vi "Anytime D Star Plan.vi"(6 "epsilon":dbl=1.0, 7 "overhaul (F)":bool, 8 "error in (no error)":errorcluster, 9 "new goal reference":refnum<data-value>, 10 "current reference":refnum<data-value>, 11 "Anytime D* in":refnum<class "NI_Robotics_AnytimeDStar.lvclass">) -> (0 "error out":errorcluster, 1 "no valid path exists":bool, 2 "path references":refnum<data-value>[](array[refnum]), 3 "Anytime D* out":refnum<class "NI_Robotics_AnytimeDStar.lvclass">, 4 "path cost":dbl)   [LabVIEW 2017, in "NI_Robotics_AnytimeDStar.lvclass"]
doc: "Plans a dynamic path through a map to the goal you specify. The first time this VI runs, the VI returns an initial path to a goal node within the map you specify in the Initialize AD* VI."
uses:
  <vilib>/robotics/Navigation/Anytime D Star/NI_Robotics_AnytimeDStar.lvclass
  <vilib>/robotics/Navigation/shared/MapNode/AbstractDstarNode/NI_Robotics_AbstractDstarNode.lvclass
  <vilib>/robotics/Navigation/Anytime D Star/NI_Robotics_AnytimeDStar.lvclass/NI_Robotics_AnytimeDStar.ctl
  <vilib>/robotics/Navigation/shared/WorldMap/AbstractDstarWorldMap/NI_Robotics_AbstractDstarWorldMap.lvclass
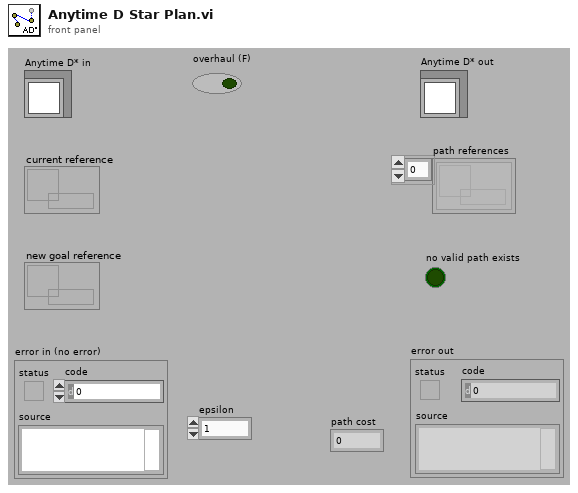
[diagram p1: front panel]
types:
  T1 = typedef "NI_Robotics_AbstractWorldMap.lvclass/World Map Edge.ctl" = cluster{"Start":refnum<data-value>, "End":refnum<data-value>, "Cost":dbl}
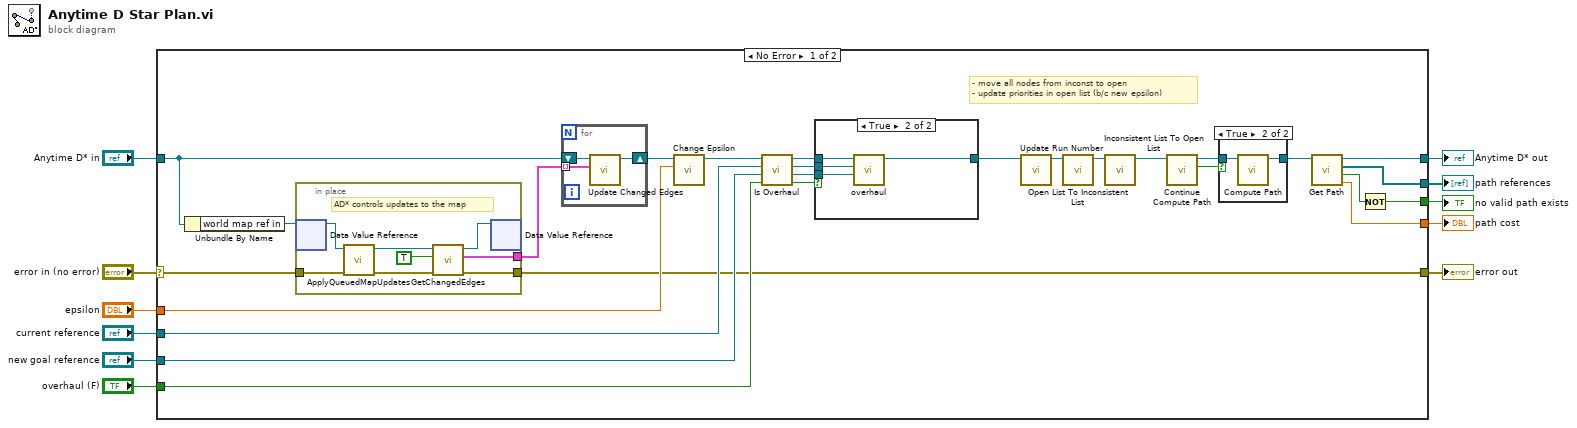
[diagram p0: block diagram]
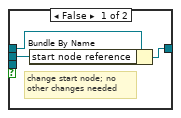
[diagram p3: hidden frame]
diagram:
  n1 = case shown="No Error" "error in (no error)" {
    selector: "error in (no error)" -> [w12 w60]
    tunnel: "Anytime D* in" -> [w38 w61]
    tunnel: "current reference" -> [w37 _]
    tunnel: "epsilon" -> [w36 _]
    tunnel: "new goal reference" -> [w35 _]
    tunnel: "overhaul (F)" -> [w34 _]
    tunnel: [w33 w61] -> w6
    tunnel: [w19 _] -> w5
    tunnel: [w18 _] -> w4
    tunnel: [w15 w60] -> w3
    tunnel: [w14 _] -> w2
    frame No Error {
      # "- move all nodes from inconst to open\n- update priorities in open list (b/c new epsilon)"
      n2 = Unbundle By Name(w38) -> ("world map ref in"=w24:refnum<data-value>)
      n3 = in-place {
        in-place-border: [w49] -> w23
        in-place-border: w12 -> [w47]
        in-place-border: [w45] -> w15
        # "AD* controls updates to the map"
        n4 = in-place-dvr #1(w24) -> (w52:refnum<class "NI_Robotics_AbstractDstarWorldMap.lvclass">)  [unwired: 1 out]
        n5 = call-dynamic "ApplyQueuedMapUpdates.vi"("error in (no error)"=w47, "AbstractWorldMap in"=w52) -> ("error out"=w46:errorcluster, "AbstractWorldMap out"=w51:refnum<class "NI_Robotics_AbstractDstarWorldMap.lvclass">)  [unwired: 8 in]
        n6 = call-dynamic "GetChangedEdges.vi"("error in (no error)"=w46, "Reset (F)"=TRUE, "AbstractWorldMap in"=w51) -> ("error out"=w45:errorcluster, "Changed Edges"=w49:T1[], "AbstractWorldMap out"=w50:refnum<class "NI_Robotics_AbstractDstarWorldMap.lvclass">)  [unwired: 6 in]
        n7 = in-place-dvr #1(w50) -> ()  [unwired: 2 out]
      }
      n8 = for {
        shift-right: [w42] -> w22
        shift-left: w38 -> [w43]
        tunnel: w23 -> [w44] mode=indexing
        n9 = call <vilib>:"Update Changed Edges.vi"("WorldMapEdge"=w44, "AD* in"=w43) -> ("AD* out"=w42:refnum<class "NI_Robotics_AnytimeDStar.lvclass">)  [unwired: 8 in, 1 out]
      }
      n10 = call <vilib>:"Change Epsilon.vi"("new epsilon"=w36, "AD* in"=w22) -> ("AD* out"=w26:refnum<class "NI_Robotics_AnytimeDStar.lvclass">)  [unwired: 9 in]
      n11 = call <vilib>:"Is Overhaul.vi"("overhaul in"=w34, "goal node in"=w35, "current node in"=w37, "AD* in"=w26) -> ("overhaul out"=w27:bool, "goal node out"=w31:refnum<data-value>, "current node out"=w32:refnum<data-value>, "AD* out"=w30:refnum<class "NI_Robotics_AnytimeDStar.lvclass">)  [unwired: 4 in]
      n12 = case shown="True" w27 {
        tunnel: [w53 w59] -> w25
        tunnel: w32 -> [w54 w58]
        tunnel: w31 -> [_ w57]
        tunnel: w30 -> [w55 w56]
        frame False {
          # "change start node; no\nother changes needed"
          n13 = Bundle By Name(cluster=w55, "start node reference"=w54) -> (w53:refnum<class "NI_Robotics_AnytimeDStar.lvclass">)
        }
        frame True {
          n14 = call <vilib>:"overhaul.vi"("goal node reference"=w57, "start node reference"=w58, "AD* in"=w56) -> ("AD* out"=w59:refnum<class "NI_Robotics_AnytimeDStar.lvclass">)  [unwired: 8 in]
        }
      }
      n15 = call <vilib>:"Update Run Number.vi"("AD* in"=w25) -> ("AD* out"=w28:refnum<class "NI_Robotics_AnytimeDStar.lvclass">)  [unwired: 10 in]
      n16 = call <vilib>:"Open List To Inconsistent List.vi"("AD* in"=w28) -> ("AD* out"=w29:refnum<class "NI_Robotics_AnytimeDStar.lvclass">)  [unwired: 10 in]
      n17 = call <vilib>:"Inconsistent List To Open List.vi"("AD* in"=w29) -> ("AD* out"=w16:refnum<class "NI_Robotics_AnytimeDStar.lvclass">)  [unwired: 10 in]
      n18 = call <vilib>:"Continue Compute Path.vi"("AD* in"=w16) -> ("continue computing path"=w20:bool, "AD* out"=w21:refnum<class "NI_Robotics_AnytimeDStar.lvclass">)  [unwired: 9 in]
      n19 = case shown="True" w20 {
        tunnel: [w39 w41] -> w17
        tunnel: w21 -> [w39 w40]
        frame False {
        }
        frame True {
          n20 = call <vilib>:"Compute Path.vi"("AD* in"=w40) -> ("AD* out"=w41:refnum<class "NI_Robotics_AnytimeDStar.lvclass">)  [unwired: 10 in]
        }
      }
      n21 = call <vilib>:"Get Path.vi"("AD* in"=w17) -> ("path cost"=w19:dbl, "valid path"=w13:bool, "path"=w18:refnum<data-value>[], "AD* out"=w33:refnum<class "NI_Robotics_AnytimeDStar.lvclass">)  [unwired: 7 in]
      n22 = Not(x=w13) -> (.not. x?=w14:bool)
    }
    frame Error {
    }
  }
  "Anytime D* out" <- w6
  "path cost" <- w5
  "path references" <- w4
  "no valid path exists" <- w2
  "error out" <- w3
